vi "Lockin_on_pulses.vi"(1 "Reference first echo?":bool, 9 "Reference Phase":dbl format="%#_13g", 10 "Frequency":dbl, 11 "Pulses":waveform(dbl)[](array[waveform])) -> (2 "Phases":dbl[](array[numeric]), 3 "Amplitudes":dbl[](array[numeric]))   [LabVIEW 2015]
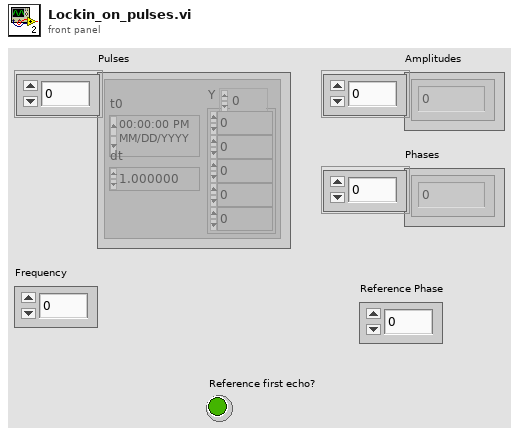
[diagram p1: front panel]
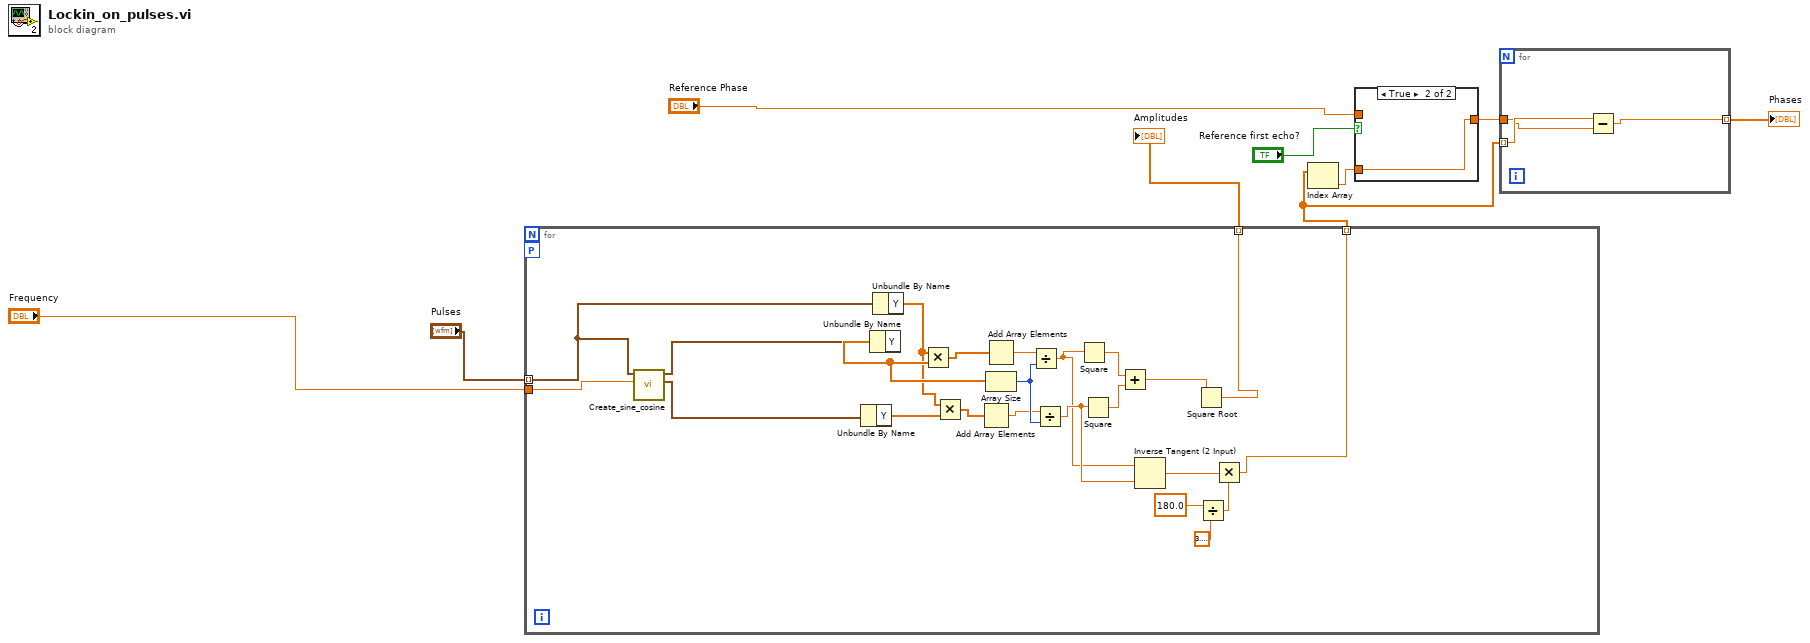
[diagram p0: block diagram]
diagram:
  n1 = for {
    tunnel: "Pulses" -> [w13] mode=indexing
    tunnel: [w15] -> w9 mode=indexing
    tunnel: "Frequency" -> [w14]
    workers-P: _ -> [_]
    tunnel: [w10] -> w3 mode=indexing
    n2 = call "Create_sine_cosine.vi"("Frequency"=w14, "Waveform Data"=w13) -> ("Cosine"=w11:waveform(dbl), "Sine"=w12:waveform(dbl))  [unwired: 8 in]
    n3 = Unbundle By Name(w11) -> ("Y"=w17:dbl[])
    n4 = Unbundle By Name(w12) -> ("Y"=w20:dbl[])
    n5 = Unbundle By Name(w13) -> ("Y"=w16:dbl[])
    n6 = Multiply(x=w16, y=w20) -> (x*y=w18:dbl[])
    n7 = Multiply(x=w16, y=w17) -> (x*y=w19:dbl[])
    n8 = Add Array Elements(numeric array=w19) -> (sum=w22:dbl)
    n9 = Add Array Elements(numeric array=w18) -> (sum=w21:dbl)
    n10 = Array Size(array=w20) -> (size(s)=w23:i32)
    n11 = Divide(x=w21, y=w23) -> (x/y=w27:dbl)
    n12 = Divide(x=w22, y=w23) -> (x/y=w28:dbl)
    n13 = Square(x=w27) -> (x^2=w24:dbl)
    n14 = Square(x=w28) -> (x^2=w25:dbl)
    n15 = Add(x=w24, y=w25) -> (x+y=w26:dbl)
    n16 = Inverse Tangent (2 Input)(1:w28, 2:w27) -> (0:w32:dbl)
    n17 = Square Root(x=w26) -> (sqrt(x)=w15:dbl)
    n18 = Divide(x=180.0, y=3.141592653589793) -> (x/y=w31:dbl)
    n19 = Multiply(x=w32, y=w31) -> (x*y=w10:dbl)
  }
  "Amplitudes" <- w9
  n20 = Index Array(array=w3) -> (element=w5:dbl)  [unwired: 1 in]
  n21 = case shown="True" "Reference first echo?" {
    tunnel: [w33 w34] -> w4
    tunnel: "Reference Phase" -> [w33 _]
    tunnel: w5 -> [_ w34]
    frame False {
    }
    frame True {
    }
  }
  n22 = for {
    tunnel: w4 -> [w36]
    tunnel: w3 -> [w37] mode=indexing
    tunnel: [w35] -> w2 mode=indexing
    n23 = Subtract(x=w37, y=w36) -> (x-y=w35:dbl)
  }
  "Phases" <- w2
